vi "Delete Files.vi"(8 "error in (no error)":errorcluster, 11 "Agent Fixture in":refnum<class "Agent Fixture.lvclass">) -> (0 "error out":errorcluster, 3 "Agent Fixture out":refnum<class "Agent Fixture.lvclass">)   [LabVIEW 2013, in "libssh2_integration_tests.lvlib" / "Agent Fixture.lvclass"]
uses:
  Agent Fixture.lvclass
  Agent Fixture.lvclass/Agent Fixture.ctl
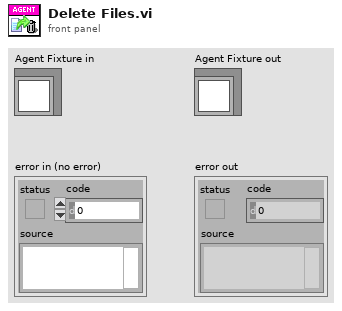
[diagram p1: front panel]
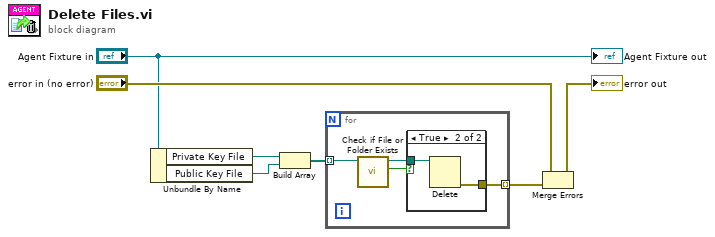
[diagram p0: block diagram]
diagram:
  n1 = Unbundle By Name("Agent Fixture in") -> ("Private Key File"=w7:path, "Public Key File"=w1:path)
  n2 = Build Array(w7, w1) -> (w6:path[])
  n3 = for {
    tunnel: [w11] -> w5 mode=indexing
    tunnel: w6 -> [w10] mode=indexing
    n4 = call <vilib>:"Check if File or Folder Exists.vi"("path"=w10) -> ("file or folder exists?"=w8:bool, "dup path"=w9:path)  [unwired: 8 in, 1 out]
    n5 = case shown="True" w8 {
      tunnel: [_ w13] -> w11
      tunnel: w9 -> [_ w12]
      frame False {
      }
      frame True {
        n6 = Delete(path (use dialog)=w12) -> (error out=w13:errorcluster)  [unwired: 4 in, 2 out]
      }
    }
  }
  n7 = Merge Errors("error in (no error)", w5) -> (→"error out":errorcluster)
  "Agent Fixture out" <- "Agent Fixture in"
